vi "set output trigger period.vi"(8 "error in (no error)":errorcluster, 11 "DAQOrcaFlash in":refnum<class "DAQOrcaFlash.lvclass">) -> (0 "error out":errorcluster, 3 "DAQOrcaFlash out":refnum<class "DAQOrcaFlash.lvclass">)   [LabVIEW 2012, in "DAQOrcaFlash.lvclass"]
uses:
  DAQOrcaFlash.lvclass
  DAQOrcaFlash.lvclass/DAQOrcaFlash.ctl
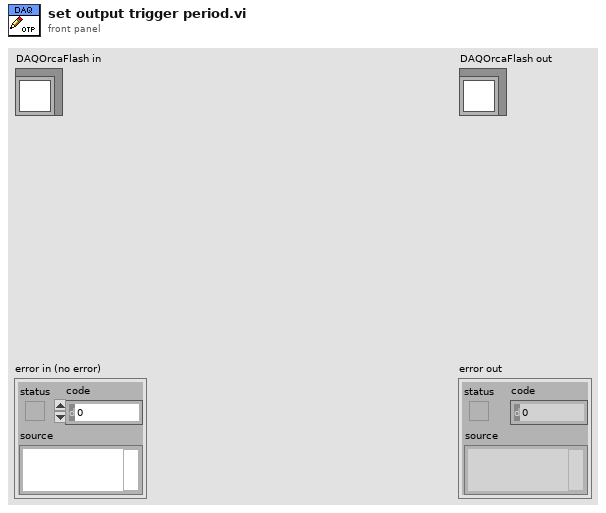
[diagram p1: front panel]
types:
  T1 = typedef "DAQOrcaFlash.lvclass/connector.ctl" = enum32{"1", "2", "3"}
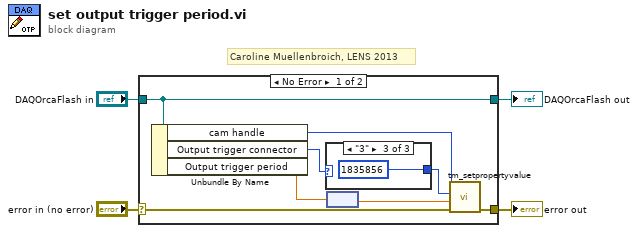
[diagram p0: block diagram]
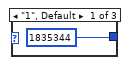
[diagram p2: hidden frame]
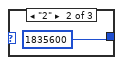
[diagram p3: hidden frame]
diagram:
  # "Caroline Muellenbroich, LENS 2013"
  n1 = case shown="No Error" "error in (no error)" {
    selector: "error in (no error)" -> [w9 w17]
    tunnel: [w8 w17] -> w3
    tunnel: [w12 w16] -> w1
    tunnel: "DAQOrcaFlash in" -> [w12 w16]
    frame No Error {
      n2 = Unbundle By Name(w12) -> ("cam handle"=w10:u32, "Output trigger connector"=w11:T1, "Output trigger period"=w7:sgl[unit])
      n3 = case shown="\"3\"" w11 {
        tunnel: [u32 1835344 ("Property ID") u32 1835600 ("Property ID") u32 1835856 ("Property ID")] -> w6
        frame "1", Default {
        }
        frame "2" {
        }
        frame "3" {
        }
      }
      n4 = node(w7) -> (w5:sgl)
      n5 = call <userlib>:"tm_setpropertyvalue.vi"("error in (no error)"=w9, "Value in"=w5, "Property ID"=w6, "Handle in"=w10) -> ("error out"=w8:errorcluster)  [unwired: 6 in, 1 out]
    }
    frame Error {
    }
  }
  "error out" <- w3
  "DAQOrcaFlash out" <- w1
